vi "1_Celsius_To_Fahrenheit(Training).vi"() -> ()   [LabVIEW 2023]
uses:
  <vilib>/Ngene/Deep Learning Toolkit/Toolkit/NN_Train/Controls/NN_Train_Params.ctl
  <vilib>/Ngene/Deep Learning Toolkit/Toolkit/NN_Train/Controls/NN_Train_Optimizer.ctl
  <vilib>/Ngene/Deep Learning Toolkit/Toolkit/NN_Train/Controls/NN_Train_Data_Sampling.ctl
  <vilib>/Ngene/Deep Learning Toolkit/Toolkit/NN_Train/Controls/NN_LR_Policy_Cfg.ctl
  <vilib>/Ngene/Deep Learning Toolkit/Toolkit/NN_Train/Controls/NN_LR_Policy_Type.ctl
  <vilib>/Ngene/Deep Learning Toolkit/Toolkit/NN_Train/Controls/NN_Train_Session_Data.ctl
  <vilib>/Ngene/Deep Learning Toolkit/Toolkit/NN_Data/API/DataSet_Types/NN_DataSet(In1D_Out1D).ctl
  <vilib>/Ngene/Deep Learning Toolkit/Toolkit/NN_Data/API/DataRef_Types/NN_Data_ref(2D_SGL).ctl
  <vilib>/Ngene/Deep Learning Toolkit/Toolkit/NN_Layers/Layers/Input/Controls/NN_Layer_Config(Input1D).ctl
  <vilib>/Ngene/Deep Learning Toolkit/Toolkit/NN_Layers/Layers/FC/Controls/NN_Layer_Config(FC).ctl
  <vilib>/Ngene/Deep Learning Toolkit/Toolkit/NN_Layers/Layers/BatchNorm/Controls/NN_BN_Params.ctl
  <vilib>/Ngene/Deep Learning Toolkit/Toolkit/NN_Activations/Controls/NN_Activation_Type.ctl
  <vilib>/Ngene/Deep Learning Toolkit/Toolkit/NN_Layers/Controls/NN_Layer_Init_Params.ctl
  <vilib>/Ngene/Deep Learning Toolkit/Toolkit/NN_Layers/Controls/NN_Layer_Weight_Init_Type.ctl
  <vilib>/Ngene/Deep Learning Toolkit/Toolkit/NN_Layers/Layers/Input/NN_Layer_Create(Input1D).vi
  <vilib>/Ngene/Deep Learning Toolkit/Toolkit/NN_Layers/Layers/FC/NN_Layer_Create(FC).vi
  <vilib>/Ngene/Deep Learning Toolkit/Toolkit/NN_Train/Loss_Functions/NN_Set_Loss(MSE).vi
  <vilib>/Ngene/Deep Learning Toolkit/Toolkit/Deep_Learning_Toolkit_by_Ngene.lvlib
panel:
  in  "Stop":bool
  out "Loss":sgl(graph)=1.1223165e-09
  out "Loss Value":sgl=1.1223165e-09 format="%#_3g"
  out "Session Data":T1={"Epochs"=2971.2, "Tot_Iter"=7428, "LR"=0.002, "LR_iter"=1}
  in  "LR_Decay_Params":T2={"Policy_Type"=enum."Manual", "LR0"=0.002, "k"=0.0, "WarmUp_Policy"=enum."Step", "WarmUp_Iter"=100, "WarmUp_Ratio"=10.0} {"WarmUp_Ratio" min=1; "WarmUp_Iter" min=1; "LR0" format="%.7f"}
  in  "NN_Train_Params":T4={"Optimizer"=enum."SGD", "Beta_1"=0.9, "Beta_2"=0.0, "Weight Decay(L1)"=1e-08, "Weight Decay(L2)"=1e-08, "Data_Sampling"=enum."Sequential"}
  # "Overview: Demonstrates the usage of Deep Learning Toolkit for solving a Celius to Fahrenheit (C2F) convertion problem.\nRequirements: DeepLTK - Deep Learning Toolkit for LabVIEW (https://www.ngene.co/deep-learning-toolkit-for-labview)\nInstructions:\n1. Run the VI.\n2. Observe how the training loss is decreasing.\n3. Observe the training speed.\n4. Press the Stop Train button when the curve stops decreasing.\nMore Examples:  https://github.com/ngenehub/deepltk_examples"
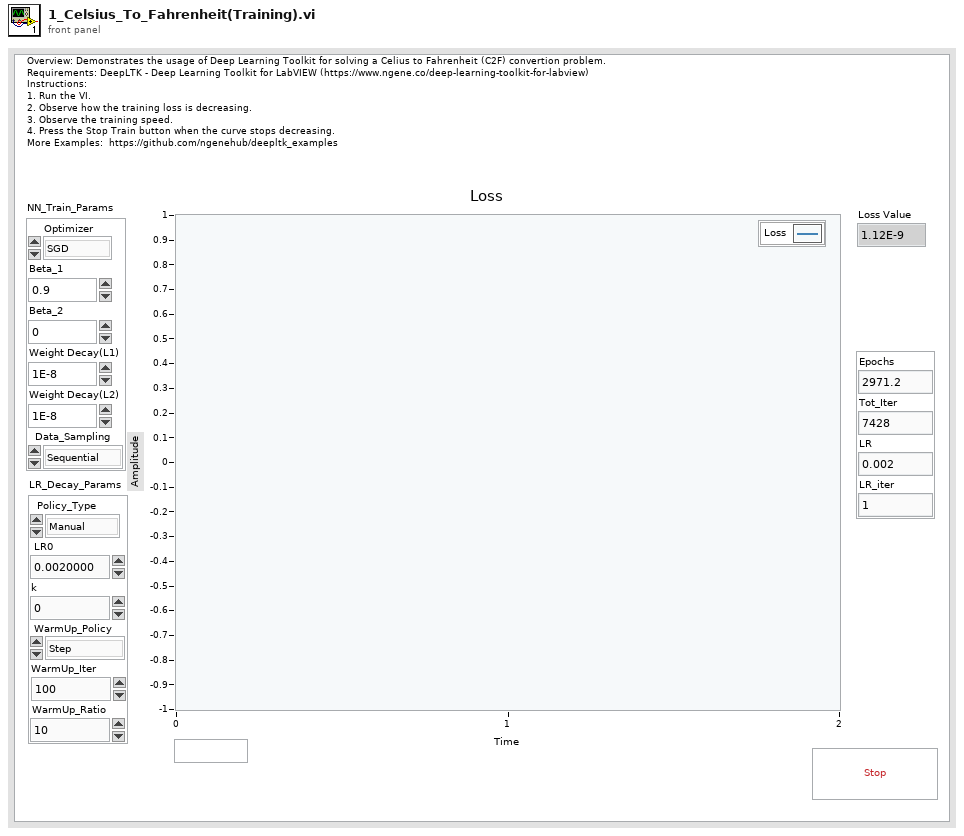
[diagram p1: front panel]
types:
  T1 = typedef "Deep_Learning_Toolkit_by_Ngene.lvlib/NN_Train_Session_Data.ctl" = cluster{"Epochs":sgl, "Tot_Iter":i32, "LR":sgl, "LR_iter":i32}
  T2 = typedef "Deep_Learning_Toolkit_by_Ngene.lvlib/NN_LR_Policy_Cfg.ctl" = cluster{"Policy_Type":T3, "LR0":dbl, "k":sgl, "WarmUp_Policy":enum16{"Step", "Ramp"}, "WarmUp_Iter":i32, "WarmUp_Ratio":sgl}
  T3 = typedef "Deep_Learning_Toolkit_by_Ngene.lvlib/NN_LR_Policy_Type.ctl" = enum16{"Manual", "Step", "Exp", "1/t"}
  T4 = typedef "Deep_Learning_Toolkit_by_Ngene.lvlib/NN_Train_Params.ctl" = cluster{"Optimizer":T5, "Beta_1":sgl, "Beta_2":sgl, "Weight Decay(L1)":sgl, "Weight Decay(L2)":sgl, "Data_Sampling":T6}
  T5 = typedef "Deep_Learning_Toolkit_by_Ngene.lvlib/NN_Train_Optimizer.ctl" = enum16{"SGD", "Adam", "Adagrad", "Adadelta", "RMSProp", "Nesterov"}
  T6 = typedef "Deep_Learning_Toolkit_by_Ngene.lvlib/NN_Train_Data_Sampling.ctl" = enum16{"Random", "Sequential"}
  T7 = typedef "Deep_Learning_Toolkit_by_Ngene.lvlib/NN_Layer_Config(FC).ctl" = cluster{"Name":string, "Size":i32, "BN":bool, "BN_Params":T8, "Activation":T9, "Has Bias?":bool, "Init_Params":T10, "Custom_Params":string}
  T8 = typedef "Deep_Learning_Toolkit_by_Ngene.lvlib/NN_BN_Params.ctl" = cluster{"epsilon":sgl, "momentum":sgl}
  T9 = typedef "Deep_Learning_Toolkit_by_Ngene.lvlib/NN_Activation_Type.ctl" = enum16{"Sigmoid", "ReLU", "LReLU", "ReLU6", "tanh", "Swish", "Mish", "None"}
  T10 = typedef "Deep_Learning_Toolkit_by_Ngene.lvlib/NN_Layer_Init_Params.ctl" = cluster{"Init_Type":T11, "Value":sgl}
  T11 = typedef "Deep_Learning_Toolkit_by_Ngene.lvlib/NN_Layer_Weight_Init_Type.ctl" = enum16{"Const", "Uniform", "Gaussian", "Xavier"}
  T12 = typedef "Deep_Learning_Toolkit_by_Ngene.lvlib/NN_Layer_Config(Input1D).ctl" = cluster{"Name":string, "Size":i32}
  T13 = typedef "Deep_Learning_Toolkit_by_Ngene.lvlib/NN_DataSet(In1D_Out1D).ctl" = cluster{"Inputs Ref.":T14, "Outputs Ref.":T14, "Dims_In":i32, "Dataset_Size":i32, "Dims_Out":i32, "Labels":string[], "File Paths":path[]}
  T14 = typedef "Deep_Learning_Toolkit_by_Ngene.lvlib/NN_Data_ref(2D_SGL).ctl" = refnum<data-value>
  T15 = typedef "Deep_Learning_Toolkit_by_Ngene.lvlib/NN.ctl" = cluster{"Name":string, "No of Layers":i32, "mBatch":i32, "Layers":T16[], "Dimty":T17, "Dims_In":T18, "Dims_Out":T18, "Working_Dir":path, "Train?":bool, "Train_Params":T4, "LR_Update_Policy":T2, "Session Data":T1, "Ground_truth":T19, "NNg_hdls":T20, "NN_Device":T21, "GPU Id":i32, "Labels":string[], "Receptive Field":T22[], "Loss_Type":T23, "Loss_Cfg_Prms":variant, "NNG_WS":T24}
  T16 = typedef "Deep_Learning_Toolkit_by_Ngene.lvlib/NN_Layer_ref.ctl" = refnum<data-value>
  T17 = typedef "Deep_Learning_Toolkit_by_Ngene.lvlib/NN_In_Out_Dim-ty.ctl" = enum8{"In1D_Out1D", "In3D_Out1D", "In3D_Out3D", "In3D_OutBBox"}
  T18 = typedef "Deep_Learning_Toolkit_by_Ngene.lvlib/NN_Dims(C,H,W).ctl" = cluster{"C":i32, "H":i32, "W":i32}
  T19 = typedef "Deep_Learning_Toolkit_by_Ngene.lvlib/NN_Ground_truth.ctl" = cluster{"Y":variant}
  T20 = typedef "Deep_Learning_Toolkit_by_Ngene.lvlib/nng_cuda_handles.ctl" = cluster{"cudnn":u64, "cublas":u64, "stream":u64, "curand":u64}
  T21 = typedef "Deep_Learning_Toolkit_by_Ngene.lvlib/NN_Device.ctl" = enum16{"CPU", "GPU"}
  T22 = typedef "Deep_Learning_Toolkit_by_Ngene.lvlib/NN_Dims(V,H).ctl" = cluster{"V":i32, "H":i32}
  T23 = typedef "Deep_Learning_Toolkit_by_Ngene.lvlib/NN_Loss_Type.ctl" = enum16{"None", "MSE", "CrossEntropy", "YOLO_v2", "YOLO_v4"}
  T24 = typedef "Deep_Learning_Toolkit_by_Ngene.lvlib/NNG_WS.ctl" = cluster{"NNG_WS_Mem":T25, "Max_WS_Size":i64}
  T25 = typedef "Deep_Learning_Toolkit_by_Ngene.lvlib/NNg_WS_Mem_DVR.ctl" = refnum<data-value>
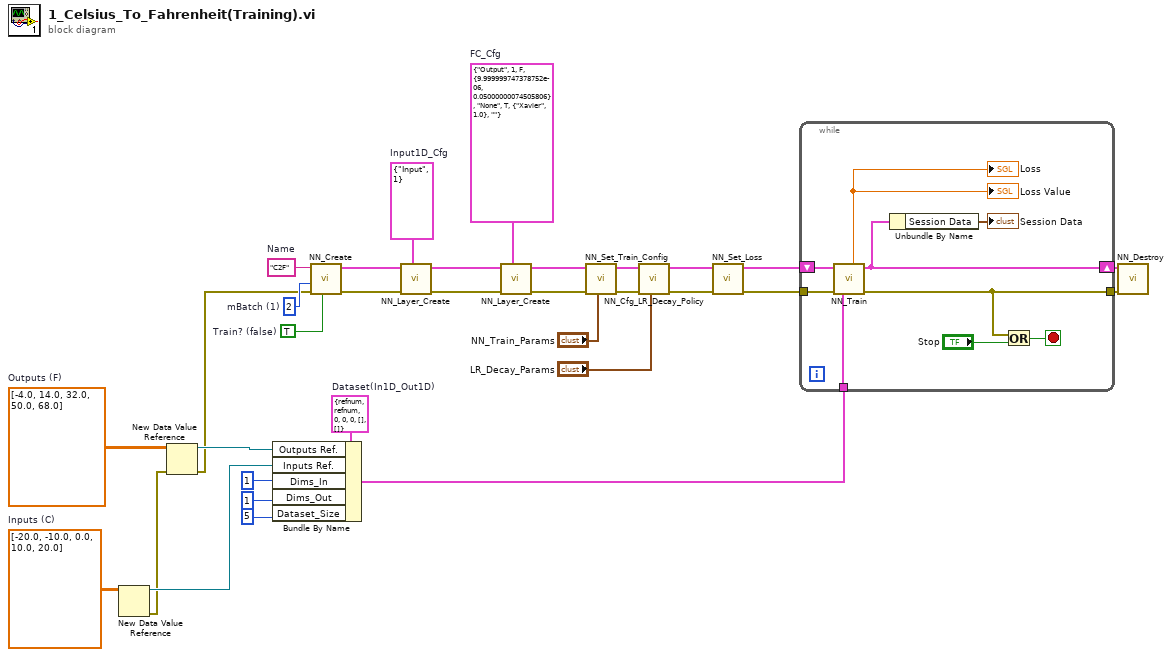
[diagram p0: block diagram]
diagram:
  w15 = 2  # mBatch (1)
  w28 = T7 {"Name"="Output", "Size"=1, "BN"=FALSE, "BN_Params"={"epsilon"=1e-05, "momentum"=0.05}, "Activation"=enum."None", "Has Bias?"=TRUE, "Init_Params"={"Init_Type"=enum."Xavier", "Value"=1.0}, "Custom_Params"=""}  # FC_Cfg
  w29 = T12 {"Name"="Input", "Size"=1}  # Input1D_Cfg
  w30 = T13 {"Inputs Ref."=refnum, "Outputs Ref."=refnum, "Dims_In"=0, "Dataset_Size"=0, "Dims_Out"=0, "Labels"=[], "File Paths"=[]}  # Dataset(In1D_Out1D)
  w31 = "C2F"  # Name
  w32 = TRUE  # Train? (false)
  w26 = sgl[][] [[-4.0], [14.0], [32.0], [50.0], [68.0]]  # Outputs (F)
  w27 = sgl[][] [[-20.0], [-10.0], [0.0], [10.0], [20.0]]  # Inputs (C)
  n1 = New Data Value Reference(data value=w27) -> (data value reference=w25:refnum<data-value>, error out=w23:errorcluster)  [unwired: 1 in]
  n2 = New Data Value Reference(data value=w26, error in=w23) -> (data value reference=w24:refnum<data-value>, error out=w9:errorcluster)
  n3 = Bundle By Name(cluster=w30, "Outputs Ref."=w24, "Inputs Ref."=w25, "Dims_In"=1, "Dims_Out"=1, "Dataset_Size"=5) -> (w4:T13)
  n4 = call <vilib>:"NN_Create.vi"("Train? (false)"=w32, "error in (no error)"=w9, "mBatch (1)"=w15, "Name"=w31) -> ("error out"=w8:errorcluster, "NN out"=w12:T15)  [unwired: 6 in]
  n5 = call-poly <vilib>:"NN_Layer_Create.vi"("Input1D_Cfg"=w29, "error in (no error)"=w8, "NN in"=w12) -> ("error out"=w7:errorcluster, "NN out"=w11:T15)  [unwired: 6 in, 1 out]
  n6 = call-poly <vilib>:"NN_Layer_Create.vi"("FC_Cfg"=w28, "error in (no error)"=w7, "NN in"=w11) -> ("error out"=w6:errorcluster, "NN out"=w10:T15)  [unwired: 6 in, 1 out]
  n7 = call <vilib>:"NN_Set_Train_Config.vi"("NN_Train_Params"="NN_Train_Params", "error in (no error)"=w6, "NN in"=w10) -> ("error out"=w20:errorcluster, "NN out"=w19:T15)  [unwired: 7 in]
  n8 = call <vilib>:"NN_Cfg_LR_Decay_Policy.vi"("LR_Decay_Params"="LR_Decay_Params", "error in (no error)"=w20, "NN in"=w19) -> ("error out"=w2:errorcluster, "NN out"=w5:T15)  [unwired: 7 in]
  n9 = call-poly <vilib>:"NN_Set_Loss.vi"("error in (no error)"=w2, "NN in"=w5) -> ("error out"=w1:errorcluster, "NN out"=w3:T15)  [unwired: 8 in]
  n10 = while {
    shift-right: [w41] -> w14
    shift-left: w3 -> [w40]
    tunnel: [w36] -> w13
    tunnel: w1 -> [w39]
    tunnel: w4 -> [w38]
    stop <- w35 stop-if-true
    n11 = call <vilib>:"NN_Train.vi"("Train Dataset"=w38, "error in (no error)"=w39, "NN in"=w40) -> ("error out"=w36:errorcluster, "NN out"=w41:T15, "Loss"=→"Loss Value" →"Loss":sgl)  [unwired: 4 in, 2 out]
    n12 = Unbundle By Name(w41) -> ("Session Data"=→"Session Data":T1)
    n13 = Or(x=w36, y="Stop") -> (x .or. y?=w35:bool)
  }
  n14 = call <vilib>:"NN_Destroy.vi"("error in (no error)"=w13, "NN in"=w14) -> ()  [unwired: 8 in, 2 out]
